vi "Slave.vi"() -> ()   [LabVIEW 2015]
uses:
  User Interface/Controls/Abort Test.ctl
  User Interface/Controls/Start Test.ctl
  User Interface/Controls/Configuration.ctl
  User Interface/Controls/Manual.ctl
  User Interface/Controls/Quit.ctl
  User Interface/UI Handler/Typedefs/Session Handle.ctl
  User Interface/UI Handler/UI Handler.lvclass
  Common/Circular Error Log/Typedefs/Session Handle.ctl
  Common/Circular Error Log/Circular Error Log.lvclass
  Tests/Controls/Test Config.ctl
  Tests/Controls/Gas Mixture.ctl
  CAN Communication/PAS/Typedefs/ADC Gains.ctl
  Tests/Controls/Filter Sequence.ctl
  Tests/Controls/Functional Test.ctl
  CAN Communication/PAS/Typedefs/Session Handle.ctl
  CAN Communication/PAS/PAS.lvclass
  Serial Device/Vaisala/Typedefs/Session Handle.ctl
  Serial Device/Vaisala/Vaisala.lvclass
  Tests/Controls/Test Info.ctl
  Serial Device/Environics/Typedefs/Session Handle.ctl
  Serial Device/Environics/Environics.lvclass
  Common/Buffers/Circular Buffer/Typedefs/Session Handle.ctl
  Common/Buffers/Circular Buffer/Circular Buffer.lvclass
  User Interface/UI Handler/Typedefs/References.ctl
  CAN Communication/PAS/Typedefs/Valves.ctl
  <vilib>/Utility/file.llb/Read Delimited Spreadsheet (string).vi
  Common/State Machine/State Machine.lvlib
  Common/Buffers/Snapshot/Snapshot.lvclass
  <vilib>/Analysis/NI_AALBase.lvlib
panel:
  in  "Quit":T1
  in  "Manual":T2
  in  "Configuration":T3
  in  "Start Test":T4
  in  "Abort Test":T5
  out "Samples Left":u16
  out "Filter Position":u8(knob) scale=1.0..12.0
  in  "Test":string
  out "PEL Temp":dbl caption="PEL Temp (C)" format="%.2f"
  out "PAS Temp":dbl caption="PAS Temp (C)" format="%.2f"
  out "Leak Rate":dbl caption="Leak Rate (PSI/s)" format="%.2f"
  out "Error?":bool
  out "Gas Stable?":bool
  out "Time Remaining":u32 caption="Time (s)"
  out "Moisture":dbl
  out "PPM":dbl caption="Actual PPM"
  out "Gas":string caption="Current Gas"
  in  "Broadcast":string
  out "exit":bool
  in  "Display":string
  out "Pressure":dbl caption="Gas Pressure (PSI)" format="%.2f"
  in  "Gas Sequence":i32(listbox)=-2
  in  "Message Log":string
  # "PAS Calibraton SLAVE"
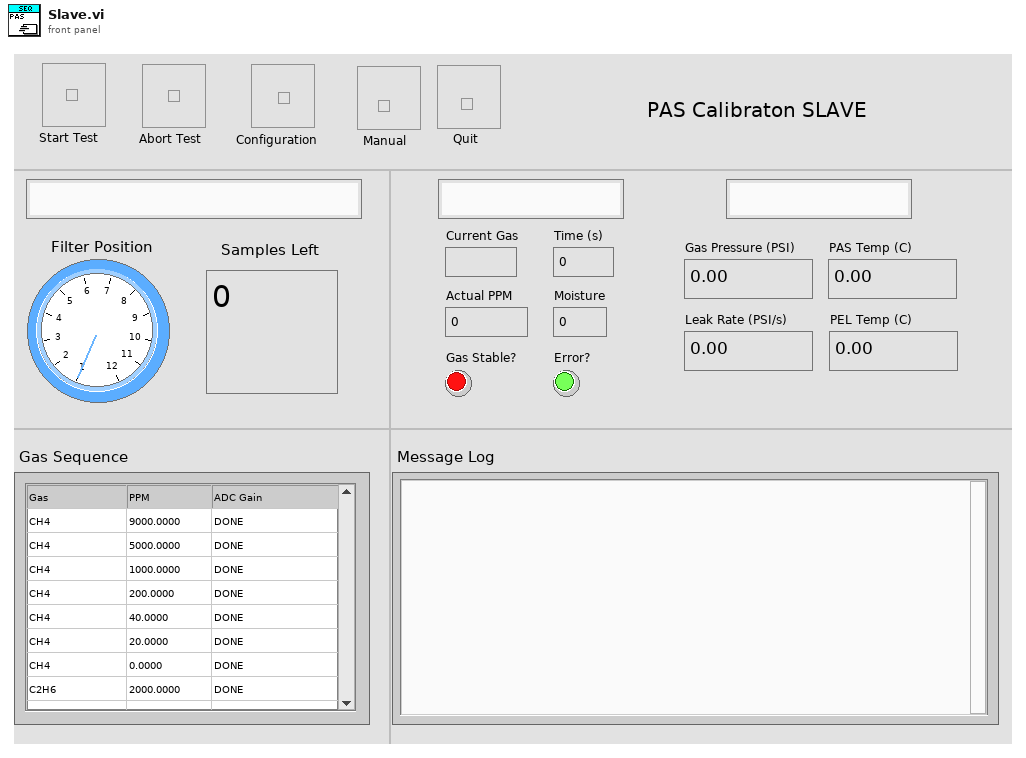
[diagram p1: front panel]
types:
  T1 = typedef "Quit.ctl" = bool
  T2 = typedef "Manual.ctl" = bool
  T3 = typedef "Configuration.ctl" = bool
  T4 = typedef "Start Test.ctl" = bool
  T5 = typedef "Abort Test.ctl" = bool
  T6 = enum8{"Enabled", "Disabled", "Disabled and Grayed Out"}
  T7 = typedef "UI Handler.lvclass/Session Handle.ctl" = refnum<data-value>
  T8 = typedef "Circular Error Log.lvclass/Session Handle.ctl" = refnum<data-value>
  T9 = typedef "Test Config.ctl" = cluster{"Chopper RPM":u16, "IR Power":u8, "Conc Tolerance":dbl, "Gas Stable Time":u16, "A-D Settle":u16, "Samples":u16, "Filter Time":u16, "Gas Mixtures":T10[], "Filter Sequences":T12[], "Functional Test":T13, "Initial Flow Rate":sgl, "Max Flow Rate":sgl}
  T10 = typedef "Gas Mixture.ctl" = cluster{"Gas":string, "PPM":dbl, "ADC Gains":T11}
  T11 = typedef "PAS.lvclass/ADC Gains.ctl" = u16
  T12 = typedef "Filter Sequence.ctl" = cluster{"Filter":u8, "Phase":dbl}
  T13 = typedef "Functional Test.ctl" = cluster{"Mic Test ON ADC Max":dbl, "Mic Test ON ADC Min":dbl, "Mic Test OFF ADC Max":dbl, "Mic Test OFF ADC Min":dbl, "Mic Test IC ADC Max":dbl, "Mic Test IC ADC Min":dbl, "IR Emitter ON ADC Max":dbl, "IR Emitter ON ADC Min":dbl, "IR Emitter OFF ADC Max":dbl, "IR Emitter OFF ADC Min":dbl}
  T14 = typedef "PAS.lvclass/Session Handle.ctl" = refnum<data-value>
  T15 = typedef "Vaisala.lvclass/Session Handle.ctl" = refnum<data-value>
  T16 = typedef "Test Info.ctl" = cluster{"Gas Counter":u16, "Filter Counter":u16, "ADC Samples":dbl[], "Gas Timeout":u16, "Notes":string, "Moisture":dbl, "PPM":dbl, "Mean":dbl, "STD":dbl, "Gas":string, "Pressure":dbl, "Temp":dbl, "Samples":u16, "Filter":u8, "Phase":dbl}
  T17 = typedef "Environics.lvclass/Session Handle.ctl" = refnum<data-value>
  T18 = typedef "Circular Buffer.lvclass/Session Handle.ctl" = refnum<data-value>
  T19 = cluster{"State":refnum<queue>, "UI Handler":T7, "Serial Number":string, "Error":T8, "Operator":string, "config path":path, "Test Config":T9, "PAS":T14, "Vaisala":T15, "Test Info":T16, "Test Results":string[][], "Environics":T17, "Cutoff":i32, "Root":path, "Circular Buffer":T18, "Zero Mean":dbl, "Zero Offsets":dbl[], "Results":T16[], "Blow Readings":cluster{"mean":dbl, "standard deviation":dbl}[], "Zero Readings":cluster{"mean":dbl, "standard deviation":dbl}[]}
  T20 = cluster{"Current Gas":string, "Actual PPM":dbl, "Moisture":dbl, "Time Remaining (s)":u32, "Stable?":bool, "Error?":bool}
  T21 = typedef "UI Handler.lvclass/References.ctl" = cluster{"Step":refnum<vi>, "Time":refnum<vi>, "Sequencer":refnum<vi>, "Log":refnum<vi>}
  T22 = cluster{"Serial Number Out":string, "Operator":string}
  T23 = typedef "PAS.lvclass/Valves.ctl" = u16
  T24 = typedef "Snapshot.lvclass/Session Handle.ctl" = refnum<data-value>
  T25 = typedef "User Configuration.ctl" = cluster{"Password":string, "cDAQ Name":string, "CAN Interface":string}
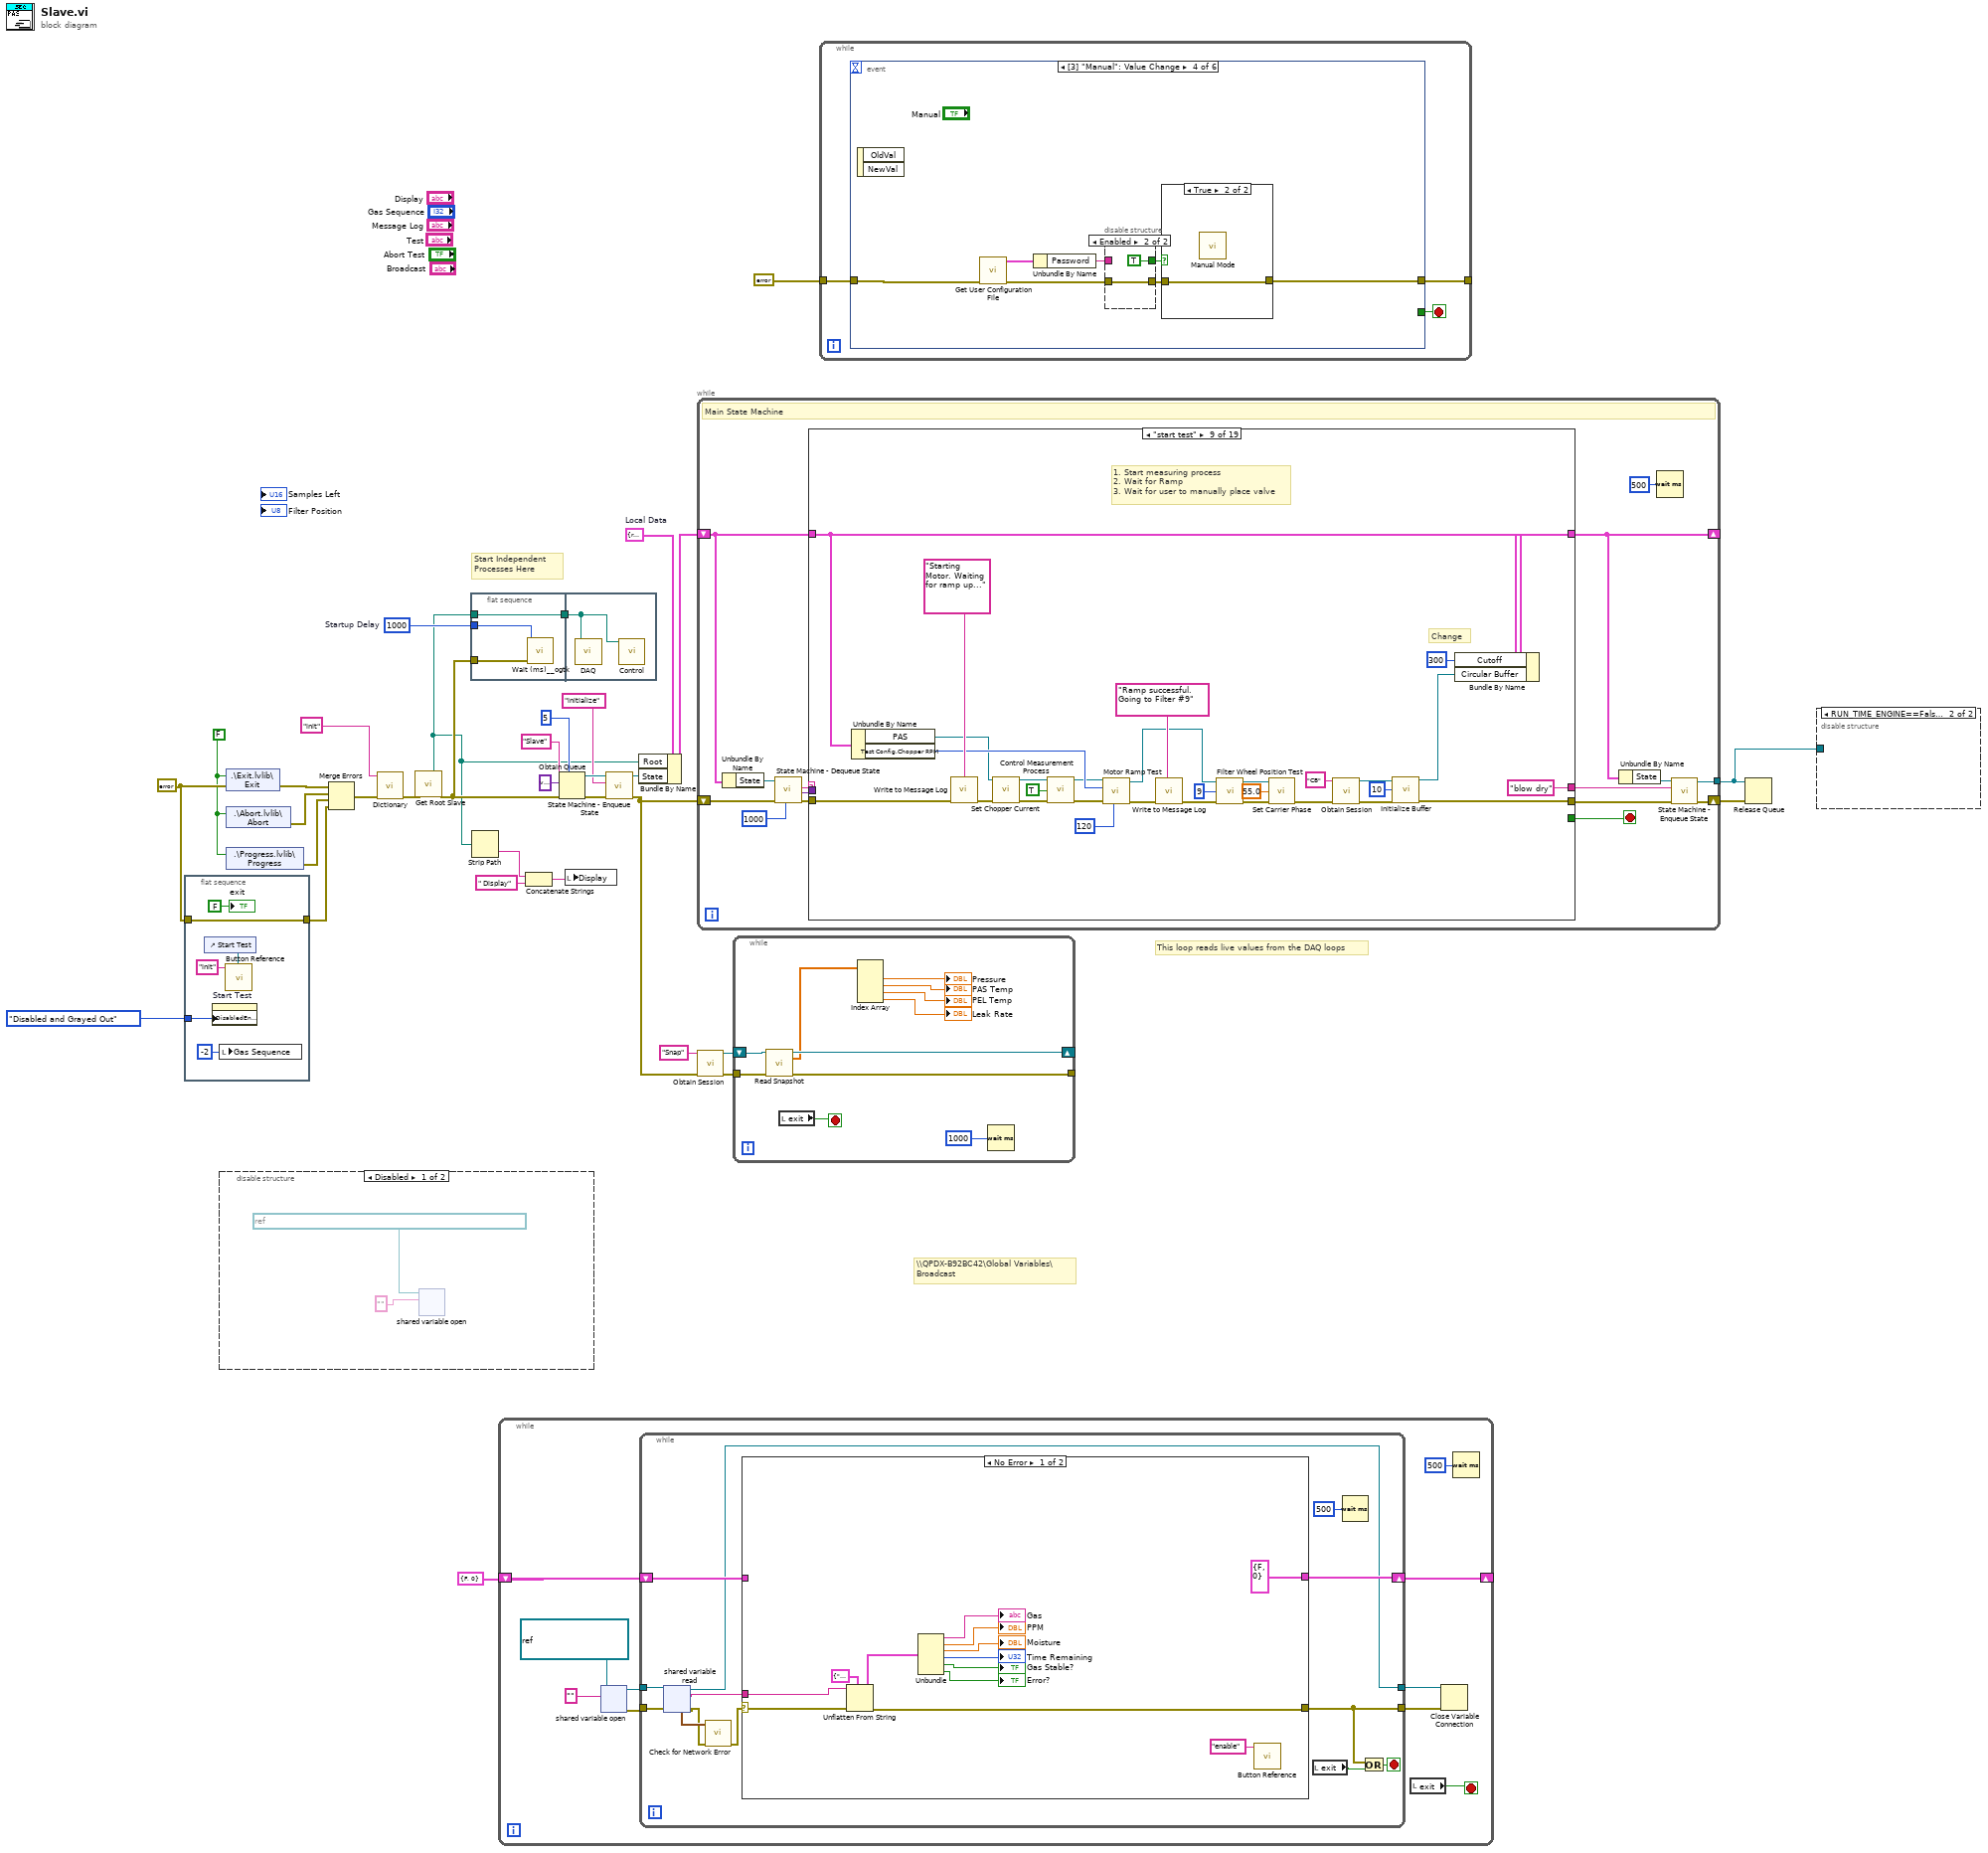
[diagram p0: block diagram]
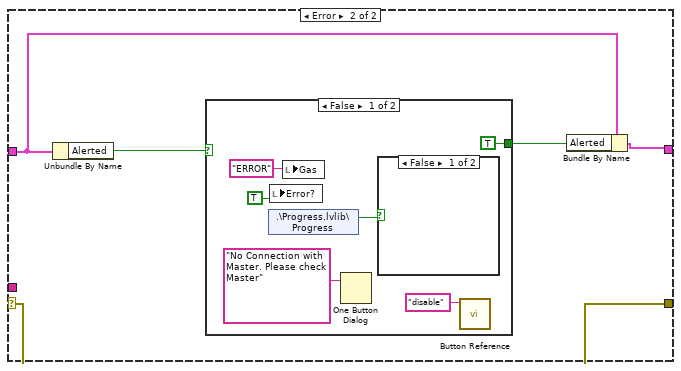
[diagram p3: hidden frame]
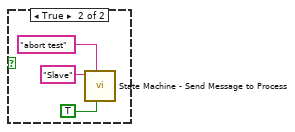
[diagram p4: hidden frame]
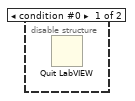
[diagram p6: hidden frame]
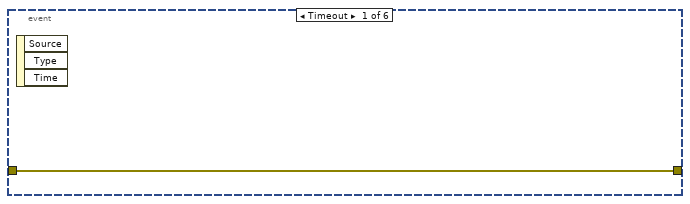
[diagram p7: hidden frame]
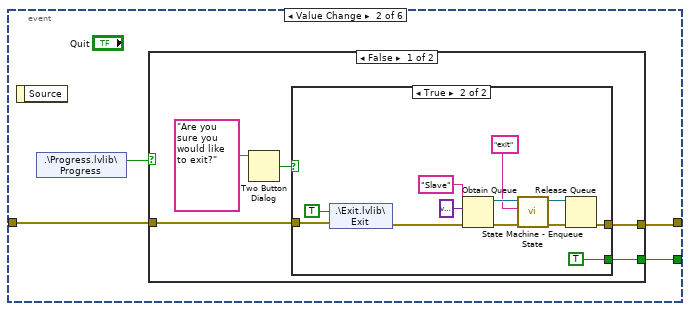
[diagram p8: hidden frame]
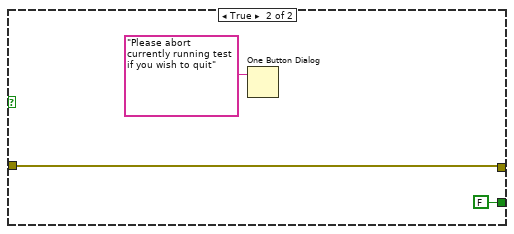
[diagram p10: hidden frame]
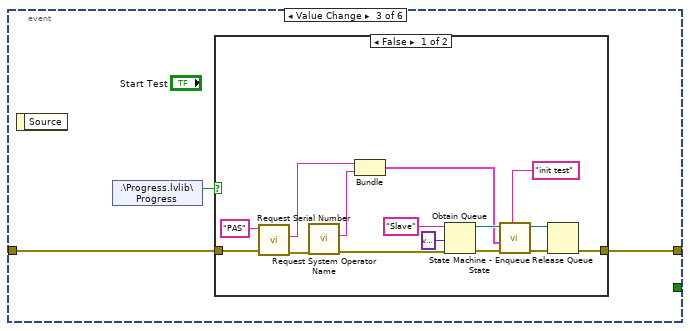
[diagram p11: hidden frame]
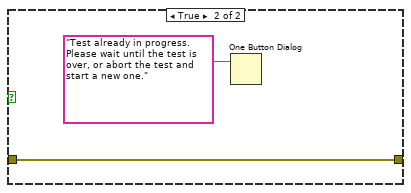
[diagram p12: hidden frame]
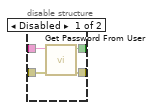
[diagram p13: hidden frame]
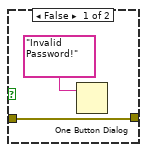
[diagram p14: hidden frame]
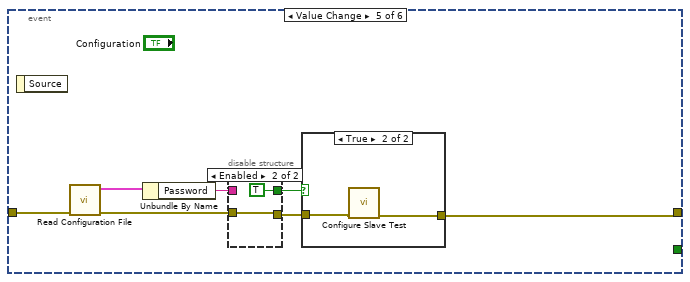
[diagram p15: hidden frame]
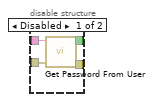
[diagram p16: hidden frame]
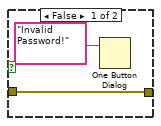
[diagram p17: hidden frame]
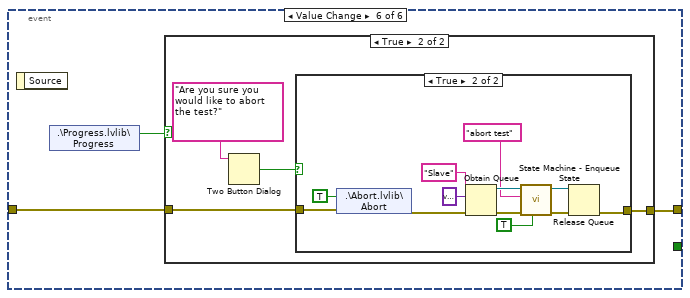
[diagram p18: hidden frame]
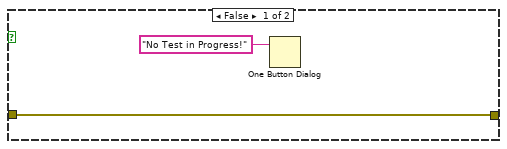
[diagram p19: hidden frame]
diagram:
  w1 = FALSE ("Exit")
  w25 = u32 1000  # Startup Delay
  w15 = errorcluster {"status"=FALSE, "code"=0, "source"=""} ("error in (no error)")
  w28 = T19 {"State"=refnum, "UI Handler"=refnum, "Serial Number"="", "Error"=refnum, "Operator"="", "config path"=path "", "Test Config"={"Chopper RPM"=140, "IR Power"=5, "Conc Tolerance"=0.0, "Gas Stable Time"=0, "A-D Settle"=0, "Samples"=0, "Filter Time"=0, "Gas Mixtures"=[], "Filter Sequences"=[], "Functional Test"={"Mic Test ON ADC Max"=0.0, "Mic Test ON ADC Min"=0.0, "Mic Test OFF ADC Max"=0.0, "Mic Test OFF ADC Min"=0.0, "Mic Test IC ADC Max"=0.0, "Mic Test IC ADC Min"=0.0, "IR Emitter ON ADC Max"=0.0, "IR Emitter ON ADC Min"=0.0, "IR Emitter OFF ADC Max"=0.0, "IR Emitter OFF ADC Min"=0.0}, "Initial Flow Rate"=0.0, "Max Flow Rate"=0.0}, "PAS"=refnum, "Vaisala"=refnum, "Test Info"={"Gas Counter"=0, "Filter Counter"=0, "ADC Samples"=[], "Gas Timeout"=0, "Notes"="", "Moisture"=0.0, "PPM"=0.0, "Mean"=0.0, "STD"=0.0, "Gas"="", "Pressure"=0.0, "Temp"=0.0, "Samples"=0, "Filter"=0, "Phase"=0.0}, "Test Results"=[], "Environics"=refnum, "Cutoff"=0, "Root"=path "", "Circular Buffer"=refnum, "Zero Mean"=0.0, "Zero Offsets"=[], "Results"=[], "Blow Readings"=[], "Zero Readings"=[]}  # Local Data
  # "\\\\QPDX-B92BC42\\Global Variables\\\nBroadcast"
  # "This loop reads live values from the DAQ loops"
  # "Start Independent\nProcesses Here"
  n1 = flat-sequence {
    tunnel: w15 -> [w39]
    tunnel: [w39] -> w14
    tunnel: T6."Disabled and Grayed Out" ("Disabled") -> [w36]
    frame #0 {
      n2 = control-ref of="Start Test"() -> (w37:refnum<vi>)
      n3 = property on="Start Test" class="Bool"("DisabledEnum"=w36) -> ()  [unwired: 2 in, 2 out]
      n4 = local write "Gas Sequence"(-2 ("Gas Sequence")) -> ()
      n5 = call "Button Reference.vi"("Ref In"=w37, "Command"="init") -> ()  [unwired: 9 in, 1 out]
      "exit" <- FALSE ("exit")
    }
  }
  n6 = disable-structure shown="Disabled" {
    frame Disabled {
      n7 = shared-variable-open(refnum<k21> "ni.var.psp://QPDX-B92BC42/Global Variables/Broadcast" ("shared variable refnum in"), "") -> ()  [unwired: 2 in, 2 out]
    }
    frame Enabled {
    }
  }
  n8 = shared-variable ".\\Exit.lvlib\\Exit"(w1, error in=w15) -> (error out=w23:errorcluster)
  n9 = shared-variable ".\\Abort.lvlib\\Abort"(w1) -> (error out=w24:errorcluster)  [unwired: 1 in]
  n10 = shared-variable ".\\Progress.lvlib\\Progress"(w1) -> (error out=w20:errorcluster)  [unwired: 1 in]
  n11 = Merge Errors(w23, w24, w20, w14) -> (w4:errorcluster)
  n12 = call "Dictionary.vi"("error in"=w4, "Command"="init") -> ("error out"=w3:errorcluster)  [unwired: 8 in, 1 out]
  n13 = call "Get Root Slave.vi"("error in (no error)"=w3) -> ("error out"=w10:errorcluster, "Root"=w5:path)  [unwired: 9 in]
  n14 = flat-sequence {
    tunnel: w10 -> [w43]
    tunnel: w25 -> [w45]
    tunnel: w5 -> [w44]
    tunnel: [w44] -> w9
    tunnel: w9 -> [w46]
    frame #0 {
      n15 = call <userlib>:"Wait (ms)__ogtk.vi"("error in (no error)"=w43, "milliseconds to wait"=w45) -> ()  [unwired: 8 in, 2 out]
    }
    frame #1 {
      n16 = call "DAQ.vi"("Folder"=w46) -> ()  [unwired: 11 in]
      n17 = call "Control.vi"("Root"=w46) -> ()  [unwired: 11 in]
    }
  }
  n18 = Strip Path(path=w5) -> (name=w8:string)  [unwired: 1 out]
  n19 = while {
    shift-right: [w53] -> _
    shift-left: cluster{"Alerted":bool, "Packets Lost":i32} {"Alerted"=FALSE, "Packets Lost"=0} -> [w54]
    stop <- w56 stop-if-true
    n20 = shared-variable-open(refnum<k21> "ni.var.psp://localhost/Global Variables/Broadcast" ("shared variable refnum in"), "") -> (w50:refnum<k21>, w51:errorcluster)  [unwired: 2 in]
    n21 = while {
      tunnel: w50 -> [w63]
      tunnel: [w61] -> w48
      tunnel: w51 -> [w64]
      tunnel: [w68] -> w49
      shift-right: [w65] -> w53
      shift-left: w54 -> [w66]
      stop <- w69 stop-if-true
      # "UDP Receiver Loop"
      n22 = shared-variable-read(w63, w64) -> (w61:refnum<k21>, w59:errorcluster, w62:string, w60:timestamp)
      n23 = call "Check for Network Error.vi"("error in (no error)"=w59, "Time Stamp"=w60) -> ("error out"=w58:errorcluster)  [unwired: 9 in]
      n24 = case shown="No Error" w58 {
        selector: w58 -> [w82 w84]
        tunnel: w62 -> [w81 _]
        tunnel: [w79 w84] -> w68
        tunnel: w66 -> [_ w85]
        tunnel: [cluster{"Alerted":bool, "Packets Lost":i32} {"Alerted"=FALSE, "Packets Lost"=0} w87] -> w65
        frame No Error {
          # "Sender sent data. Update the chart value."
          n25 = Unflatten From String(type=T20 {"Current Gas"="", "Actual PPM"=0.0, "Moisture"=0.0, "Time Remaining (s)"=0, "Stable?"=FALSE, "Error?"=FALSE} ("output cluster"), binary string=w81, error in (no error)=w82) -> (value=w78:T20, error out=w79:errorcluster)  [unwired: 2 in, 1 out]
          n26 = Unbundle(w78) -> ("Current Gas"=→"Gas":string, "Actual PPM"=→"PPM":dbl, "Moisture"=→"Moisture":dbl, "Time Remaining (s)"=→"Time Remaining":u32, "Stable?"=→"Gas Stable?":bool, "Error?"=→"Error?":bool)
          n27 = call "Button Reference.vi"("Command"="enable") -> ()  [unwired: 10 in, 1 out]
        }
        frame Error {
          # "Sender did not send data. Ignore timeout error and keep waiting."
          n28 = Unbundle By Name(w85) -> ("Alerted"=w86:bool)
          n29 = case shown="False" w86 {
            selector: w86 -> [_ w97]
            tunnel: [TRUE w97] -> w83
            frame False {
              n30 = shared-variable ".\\Progress.lvlib\\Progress"() -> (w93:bool)  [unwired: 1 in, 1 out]
              n31 = local write "Error?"(TRUE ("Error?")) -> ()
              n32 = local write "Gas"("ERROR" ("Gas")) -> ()
              n33 = One Button Dialog(message="No Connection with Master. Please check Master") -> ()  [unwired: 1 in, 1 out]
              n34 = case shown="False" w93 {
                frame False {
                }
                frame True {
                  n35 = call "State Machine - Send Message to Process.vi"("Front?"=TRUE, "State"="abort test", "Process Name"="Slave") -> ()  [unwired: 8 in, 1 out]
                }
              }
              n36 = call "Button Reference.vi"("Command"="disable") -> ()  [unwired: 10 in, 1 out]
            }
            frame True {
            }
          }
          n37 = Bundle By Name(cluster=w85, "Alerted"=w83) -> (w87:cluster{"Alerted":bool, "Packets Lost":i32})
        }
      }
      n38 = local read "exit"() -> (w67:bool)
      n39 = Wait (ms)(milliseconds to wait=u32 500) -> ()  [unwired: 1 out]
      n40 = Or(x=w68, y=w67) -> (x .or. y?=w69:bool)
    }
    n41 = local read "exit"() -> (w56:bool)
    n42 = Close Variable Connection(8:w49, 11:w48) -> ()  [unwired: 1 out]
    n43 = Wait (ms)(milliseconds to wait=u32 500) -> ()  [unwired: 1 out]
  }
  n44 = Concatenate Strings(w8, " Display" ("string")) -> (w6:string)
  n45 = Obtain Queue(max queue size (-1, unlimited)=5, name (unnamed)="Slave", element data type=variant, error in (no error)=w10) -> (queue out=w30:refnum<queue>, error out=w31:errorcluster)  [unwired: 1 in, 1 out]
  n46 = local write "Display"(w6) -> ()
  n47 = call "State Machine - Enqueue State.vi"("error in (no error)"=w31, "State"="initialize", "Queue In"=w30) -> ("error out"=w18:errorcluster, "Queue Out"=w27:refnum<queue>)  [unwired: 7 in]
  n48 = Bundle By Name(cluster=w28, "Root"=w5, "State"=w27) -> (w26:T19)
  n49 = while "Main State Machine" {
    shift-right: [w109] -> w21
    shift-left: w18 -> [w112]
    shift-right: [w100] -> _
    shift-left: w26 -> [w103]
    tunnel: [w98] -> w13
    stop <- w105 stop-if-true
    # "Main State Machine"
    n50 = Unbundle By Name(w103) -> ("State"=w102:refnum<queue>)
    n51 = call "State Machine - Dequeue State.vi"("Timeout"=1000, "error in (no error)"=w112, "Queue In"=w102) -> ("error out"=w111:errorcluster, "Data"=w99:variant, "State"=w110:string)  [unwired: 4 in, 2 out]
    n52 = case shown="\"start test\"" w110 {
      tunnel: w111 -> [w124 w150 w164 w188 w190 _ w232 w266 w288 w302 w335 w377 w409 w443 w497 w516 w546 w555 w580]
      tunnel: [w138 w147 w168 w188 w190 w195 w211 w261 w281 w306 w330 w381 w403 w439 w493 w512 w539 w551 w577] -> w108
      tunnel: ["init local" ("State") _ _ _ _ _ w226 "start test" ("Error String") "blow dry" ("Error String") w307 w343 "filter" ("Error String") w410 w440 "start mix" ("Error String") "record result" ("Error String") "filter" ("Error String") _ _] -> w107
      tunnel: [_ _ _ _ _ TRUE _ _ _ _ _ _ _ _ _ _ _ _ _] -> w105
      tunnel: w103 -> [w114 w157 w161 w187 w189 w198 w229 w265 w287 w303 w342 w399 w408 w435 w499 w520 w549 w569 w576]
      tunnel: [w143 w157 w166 w187 w189 w198 w230 w264 w286 w303 w336 w398 w408 w434 w499 w519 w548 w569 w576] -> w100
      tunnel: w99 -> [_ _ _ _ _ _ w231 _ _ _ _ _ _ _ _ _ _ _ _]
      frame "initialize" {
        # "1. Setup UI Handler\n2. Setup Error Logger\n3. Get list of gases"
        n53 = Unbundle By Name(w114) -> ("Root"=w113:path)
        n54 = Build Path(base path=w113, name or relative path="Configuration\\Gases.txt") -> (appended path=w123:path)
        n55 = call-poly <vilib>:"Read Delimited Spreadsheet.vi"("file path (dialog if empty)"=w123, "error in (no error)"=w124, "delimiter (\\t)"="\r") -> ("all rows"=w117:string[][], "error out"=w121:errorcluster)  [unwired: 7 in, 4 out]
        n56 = Index Array(array=w117, index (col)=0 ("disabled index (col)")) -> (element=w116:string[])  [unwired: 1 in]
        n57 = control-ref of="Gas Sequence"() -> (w128:refnum<vi>)
        n58 = call "Dictionary.vi"("error in"=w121, "Value"=w116, "Key"="Gas", "Command"="set") -> ("error out"=w118:errorcluster)  [unwired: 6 in, 1 out]
        n59 = control-ref of="Message Log"() -> (w127:refnum<vi>)
        n60 = Bundle By Name(cluster=T21 {"Step"=refnum, "Time"=refnum, "Sequencer"=refnum, "Log"=refnum} ("References"), "Sequencer"=w128, "Log"=w127) -> (w126:T21)
        n61 = call "Obtain Session.vi"("Session  Name ()"="UIH", "error in (no error)"=w118) -> ("Session Handle"=w130:T7, "error out"=w133:errorcluster)  [unwired: 12 in]
        n62 = call "Initialize References.vi"("Session Handle in"=w130, "References"=w126, "error in (no error)"=w133) -> ("Session Handle out"=w131:T7, "error out"=w132:errorcluster)  [unwired: 11 in]
        n63 = Build Path(base path=w113, name or relative path="Error\\error.txt") -> (appended path=w135:path)
        n64 = call "Obtain Session.vi"("Session  Name ()"="Error", "error in (no error)"=w132) -> ("Session Handle"=w140:T8, "error out"=w141:errorcluster)  [unwired: 12 in]
        n65 = call "Initialize Error Log.vi"("Session Handle in"=w140, "Error Path"=w135, "Max File Size"=i64 5000000, "error in (no error)"=w141) -> ("Session Handle out"=w137:T8, "error out"=w138:errorcluster)  [unwired: 10 in]
        n66 = Bundle By Name(cluster=w114, "UI Handler"=w131, "Error"=w137) -> (w143:T19)
      }
      frame "init local" {
        w146 = 0.0 ("Test Pressure (PSI)")
        # "1. Set Filter Position and Samples Remaining to 20\n2. Clear Listbox and Log\n3. Set Live Display and Test to values \n4. Set Live Display values to 0"
        n67 = call "Initialize Message Log.vi"("error in (no error)"=w150) -> ("error out"=w156:errorcluster)  [unwired: 10 in]
        n68 = call "Clear Sequence.vi"("error in (no error)"=w156) -> ("error out"=w153:errorcluster)  [unwired: 10 in]
        n69 = call "Write to Message Log.vi"("error in (no error)"=w153, "Message"="PAS Calibration Started...") -> ("error out"=w145:errorcluster)  [unwired: 9 in]
        n70 = property on="Test" class="Str"(error in=w145, "Value"="No Test In Progress..." ("Test")) -> (error out=w149:errorcluster)  [unwired: 1 in, 1 out]
        n71 = property on="Broadcast" class="Str"(error in=w149, "Text.Text"="Broadcast Data...") -> (error out=w147:errorcluster)  [unwired: 1 in, 1 out]
        n72 = local write "Pressure"(w146) -> ()
        n73 = local write "PAS Temp"(w146) -> ()
        n74 = local write "PEL Temp"(w146) -> ()
        n75 = local write "Leak Rate"(w146) -> ()
        n76 = local write "Filter Position"(u8 0 ("Filter Position")) -> ()
        n77 = local write "Samples Left"(u16 0 ("Samples Left")) -> ()
      }
      frame "error" {
        # "1. If a test was in progress..."
        n78 = call "Data Changed.vi"("Data"=w164) -> ("Changed?"=w163:bool)  [unwired: 10 in]
        n79 = case shown="True" w163 {
          tunnel: [w169 w173] -> w160
          tunnel: w164 -> [w170 w174]
          frame False {
            n80 = Unbundle By Name(w170) -> ("source"=w171:string)
            n81 = Concatenate Strings("Error: " ("string"), w171) -> (w169:string)
          }
          frame True {
            n82 = Unbundle By Name(w174) -> ("source"=w175:string)
            n83 = Concatenate Strings("Error: " ("string"), w175) -> (w173:string)
            n84 = call "Dialog Box.vi"("Serial Number"=w173) -> ()  [unwired: 10 in, 1 out]
          }
        }
        n85 = Unbundle By Name(w161) -> ("Error"=w162:T8)
        n86 = call "Write to Message Log.vi"("Message"=w160) -> ()  [unwired: 10 in, 1 out]
        n87 = shared-variable ".\\Progress.lvlib\\Progress"() -> (w165:bool)  [unwired: 1 in, 1 out]
        n88 = call "Write Error Log.vi"("Session Handle in"=w162, "Process Name"="Main", "Data"=w160) -> ()  [unwired: 11 in, 2 out]
        n89 = case shown="True" w165 {
          tunnel: w161 -> [w177 w181]
          tunnel: [w177 w181] -> w166
          tunnel: w160 -> [_ _]
          frame False {
          }
          frame True {
            n90 = shared-variable ".\\Progress.lvlib\\Progress"(FALSE ("Progress")) -> (error out=w184:errorcluster)  [unwired: 1 in]
            n91 = call "Initialize Hardware.vi"("error in"=w184) -> ("error out"=w180:errorcluster)  [unwired: 10 in]
            n92 = local write "Test"("Test Error..." ("Test")) -> ()
            n93 = call "File Tracker.vi"("Command"="close", "error in (no error)"=w180) -> ("error out"=w179:errorcluster)  [unwired: 8 in, 1 out]
            n94 = flat-sequence {
              tunnel: "Error occured. Please see log for details. The test has been aborted" -> [w186]
              tunnel: w179 -> [_]
              frame #0 {
                n95 = One Button Dialog(message=w186) -> ()  [unwired: 1 in, 1 out]
              }
            }
          }
        }
        n96 = Unbundle By Name(w166) -> ("State"=w167:refnum<queue>)
        n97 = Wait (ms)(milliseconds to wait=u32 1000) -> ()  [unwired: 1 out]
        n98 = Flush Queue(queue=w167) -> (error out=w168:errorcluster)  [unwired: 1 in, 2 out]
      }
      frame Default {
      }
      frame "idle" {
      }
      frame "exit" {
        # "1. Clean up all references\n2. Exit commands to Datalogger"
        n99 = Unbundle By Name(w198) -> ("UI Handler"=w197:T7)
        n100 = call "Release Session.vi"("Session Handle"=w197) -> ("error out"=w193:errorcluster)  [unwired: 14 in]
        n101 = call "Write to Message Log.vi"("error in (no error)"=w193, "Message"="Initializing Hardware Before Exiting...") -> ("error out"=w192:errorcluster)  [unwired: 9 in]
        n102 = call "Initialize Hardware.vi"("error in"=w192) -> ("error out"=w191:errorcluster)  [unwired: 10 in]
        n103 = local write "exit"(TRUE ("exit")) -> ()
        n104 = flat-sequence {
          tunnel: [w200] -> w195
          tunnel: w191 -> [_]
          frame #0 {
            n105 = call "State Machine - Send Message to Process.vi"("Front?"=TRUE, "State"="exit", "Process Name"="DAQ") -> ("error out"=w201:errorcluster)  [unwired: 8 in]
            n106 = call "State Machine - Send Message to Process.vi"("Front?"=TRUE, "State"="exit", "error in (no error)"=w201, "Process Name"="Control") -> ("error out"=w200:errorcluster)  [unwired: 7 in]
          }
        }
      }
      frame "init test" {
        # "1. Initialize all Hardware\n2. Store Serial Number\n3. Send start command to logger\n4.. Proceed to Test"
        n107 = Variant To Data(error in=w232, type=T22 {"Serial Number Out"="", "Operator"=""} ("cluster"), Variant=w231) -> (data=w222:T22, error out=w221:errorcluster)
        n108 = call "Get Slave Configuration File from User.vi"("error in"=w221) -> ("error out"=w220:errorcluster, "Test Config"=w219:T9, "selected path"=w215:path)  [unwired: 7 in, 1 out]
        n109 = disable-structure shown="Enabled" {
          disable-tunnel: [w236 w238] -> w225
          disable-tunnel: [w235 TRUE ("Go on?")] -> w224
          disable-tunnel: w220 -> [w234 w238]
          disable-tunnel: w219 -> [w233 _]
          frame Disabled {
            n110 = call "PAS Functional Test.vi"("error in (no error)"=w234, "Test Config"=w233) -> ("Error Out"=w236:errorcluster, "Go on?"=w235:bool)  [unwired: 8 in]
          }
          frame Enabled {
          }
        }
        n111 = local write "Test"("Test In Progress..." ("Test")) -> ()
        n112 = case shown="False" w224 {
          tunnel: [w244 w247] -> w211
          tunnel: w225 -> [w244 w251]
          tunnel: [w239 w246] -> w212
          tunnel: [_ TRUE ("Progress")] -> w223
          tunnel: w222 -> [w243 w255]
          tunnel: [w241 w253] -> w216
          tunnel: w219 -> [w239 w246]
          tunnel: [w242 w254] -> w217
          tunnel: w215 -> [w240 w252]
          tunnel: [w240 w252] -> w214
          frame False {
            n113 = Unbundle By Name(w243) -> ("Operator"=w242:string, "Serial Number Out"=w241:string)
          }
          frame True {
            n114 = Unbundle By Name(w255) -> ("Operator"=w254:string, "Serial Number Out"=w253:string)
            n115 = call "Write to Message Log.vi"("error in (no error)"=w251, "Message"="Test Starting...") -> ("error out"=w250:errorcluster)  [unwired: 9 in]
            n116 = call "Write to Message Log.vi"("error in (no error)"=w250, "Message"="Initializing Hardware...") -> ("error out"=w260:errorcluster)  [unwired: 9 in]
            n117 = call "Initialize Hardware.vi"("error in"=w260) -> ("error out"=w256:errorcluster)  [unwired: 10 in]
            n118 = shared-variable ".\\Progress.lvlib\\Progress"(TRUE ("Progress"), error in=w256) -> (error out=w248:errorcluster)
            n119 = call "Test Tracker.vi"("Command"="init", "Test Config"=w246) -> ()  [unwired: 6 in, 4 out]
            n120 = call "Write Gas Sequence.vi"("error in (no error)"=w248, "Test Config"=w246) -> ("error out"=w247:errorcluster)  [unwired: 9 in]
          }
        }
        n121 = Bundle By Name(cluster=w229, "Test Info"=T16 {"Gas Counter"=0, "Filter Counter"=0, "ADC Samples"=[], "Gas Timeout"=0, "Notes"="", "Moisture"=0.0, "PPM"=0.0, "Mean"=0.0, "STD"=0.0, "Gas"="", "Pressure"=0.0, "Temp"=0.0, "Samples"=0, "Filter"=0, "Phase"=0.0}, "Operator"=w217, "Serial Number"=w216, "config path"=w214, "Test Config"=w212, "Zero Readings"=cluster{"mean":dbl, "standard deviation":dbl}[] [], "Results"=T16[] []) -> (w230:T19)
        n122 = Select(t="get refs" ("Error String"), s=w223, f="idle" ("Error String")) -> (s? t:f=w226:string)
      }
      frame "get refs" {
        # "1. Get References to PAS"
        n123 = call "Obtain Session.vi"("Session  Name ()"="PAS", "error in (no error)"=w266) -> ("Session Handle"=w263:T14, "error out"=w261:errorcluster)  [unwired: 12 in]
        n124 = Bundle By Name(cluster=w265, "PAS"=w263) -> (w264:T19)
      }
      frame "start test" {
        # "Change"
        # "1. Start measuring process\n2. Wait for Ramp\n3. Wait for user to manually place valve"
        n125 = Unbundle By Name(w287) -> ("PAS"=w271:T14, "Test Config.Chopper RPM"=w296:u16)
        n126 = call "Write to Message Log.vi"("error in (no error)"=w288, "Message"="Starting Motor. Waiting for ramp up...") -> ("error out"=w268:errorcluster)  [unwired: 9 in]
        n127 = call "Set Chopper Current.vi"("Session Handle in"=w271, "error in (no error)"=w268) -> ("Session Handle out"=w270:T14, "error out"=w269:errorcluster)  [unwired: 11 in, 1 out]
        n128 = call "Control Measurement Process.vi"("Session Handle in"=w270, "Start?"=TRUE, "error in (no error)"=w269) -> ("Session Handle out"=w290:T14, "error out"=w291:errorcluster)  [unwired: 9 in, 2 out]
        n129 = call "Motor Ramp Test.vi"("Timeout"=u32 120, "error in (no error)"=w291, "RPM"=w296, "Session Handle in"=w290) -> ("error out"=w294:errorcluster, "Session Handle out"=w277:T14)  [unwired: 5 in, 1 out]
        n130 = call "Write to Message Log.vi"("error in (no error)"=w294, "Message"="Ramp successful. Going to Filter #9") -> ("error out"=w279:errorcluster)  [unwired: 9 in]
        n131 = call "Filter Wheel Position Test.vi"("error in (no error)"=w279, "Position"=u8 9, "Session Handle in"=w277) -> ("error out"=w276:errorcluster, "Session Handle out"=w275:T14)  [unwired: 6 in, 1 out]
        n132 = call "Set Carrier Phase.vi"("Session Handle in"=w275, "Phase"=55.0, "error in (no error)"=w276) -> ("error out"=w273:errorcluster)  [unwired: 10 in, 2 out]
        n133 = call "Obtain Session.vi"("Session  Name ()"="CB", "error in (no error)"=w273) -> ("Session Handle"=w283:T18, "error out"=w284:errorcluster)  [unwired: 12 in]
        n134 = call "Initialize Buffer.vi"("Session Handle in"=w283, "Size"=u16 10, "error in (no error)"=w284) -> ("Session Handle out"=w280:T18, "error out"=w281:errorcluster)  [unwired: 11 in]
        n135 = Bundle By Name(cluster=w287, "Cutoff"=300, "Circular Buffer"=w280) -> (w286:T19)
      }
      frame "blow dry" {
        n136 = call "Dialog Box.vi"("error in (no error)"=w302, "Serial Number"="Beginning the Blow Dry process. Please turn the 3 Way Valve to the correct position...") -> ("error out"=w300:errorcluster)  [unwired: 9 in]
        n137 = call "File Tracker.vi"("Command"="new", "error in (no error)"=w300) -> ("error out"=w299:errorcluster)  [unwired: 8 in, 1 out]
        n138 = call "Write to Message Log.vi"("error in (no error)"=w299, "Message"="Conducting Blow Dry Test...") -> ("error out"=w304:errorcluster)  [unwired: 9 in]
        n139 = Unbundle By Name(w303) -> ("Circular Buffer"=w309:T18, "PAS"=w308:T14)
        n140 = disable-structure shown="Enabled" {
          disable-tunnel: w309 -> [w318 _]
          disable-tunnel: w308 -> [w317 _]
          disable-tunnel: [w313 "zero offset" ("State")] -> w307
          disable-tunnel: [w312 w326] -> w306
          disable-tunnel: w304 -> [w311 w326]
          frame Disabled {
            # "todo: add config"
            n141 = call "Blow Dry Test.vi"("Tol"=10000.0, "error in (no error)"=w311, "PAS"=w317, "Circular Buffer"=w318) -> ("error out"=w315:errorcluster, "Aborted?"=w314:bool, "Test Reading"=w310:cluster{"mean":dbl, "standard deviation":dbl})  [unwired: 4 in, 1 out]
            n142 = case shown="False" w314 {
              tunnel: w315 -> [w321 w323]
              tunnel: [w320 w323] -> w312
              tunnel: ["zero offset" ("State") "abort test" ("State")] -> w313
              tunnel: w310 -> [_ _]
              frame False {
                n143 = call "Write to Message Log.vi"("error in (no error)"=w321, "Message"="Blow Dry Test Succeeded") -> ("error out"=w320:errorcluster)  [unwired: 9 in]
              }
              frame True {
              }
            }
          }
          frame Enabled {
          }
        }
      }
      frame "zero offset" {
        # "todo: add config"
        n144 = Unbundle By Name(w342) -> ("PAS"=w341:T14)
        n145 = call "Flush Gas.vi"("Display UI?"=TRUE, "error in (no error)"=w335, "PAS"=w341) -> ("error out"=w333:errorcluster, "PAS Out"=w339:T14)  [unwired: 7 in]
        n146 = call "Write to Message Log.vi"("error in (no error)"=w333, "Message"="Conducting Zero Offset Test...") -> ("error out"=w332:errorcluster)  [unwired: 9 in]
        n147 = call "Zero Offset Test.vi"("Tol"=10000.0, "error in (no error)"=w332, "PAS"=w339) -> ("error out"=w345:errorcluster, "Aborted?"=w344:bool, "Success?"=w338:bool, "Readings"=w337:cluster{"mean":dbl, "standard deviation":dbl}[])  [unwired: 5 in]
        n148 = case shown="False" w344 {
          tunnel: w345 -> [w350 w361]
          tunnel: [w349 w361] -> w331
          tunnel: [w351 "abort test" ("State")] -> w343
          tunnel: [w346 _] -> w329
          tunnel: w338 -> [w348 _]
          tunnel: w337 -> [w347 _]
          frame False {
            n149 = case shown="True" w348 {
              tunnel: [_ "wait mix" ("State")] -> w351
              tunnel: w350 -> [w354 w359]
              tunnel: [w353 w358] -> w349
              tunnel: [w355 w356] -> w346
              tunnel: w347 -> [w355 w356]
              frame False {
                n150 = Merge Errors(w354, errorcluster {"status"=TRUE, "code"=781, "source"="Inconsistent ADC Readings for Zero Offset Test"} ("error in")) -> (w353:errorcluster)
              }
              frame True {
                n151 = call "Write to Message Log.vi"("error in (no error)"=w359, "Message"="Zero Offset Test Succeeded. Starting test...") -> ("error out"=w358:errorcluster)  [unwired: 9 in]
              }
            }
          }
          frame True {
          }
        }
        n152 = Bundle By Name(cluster=w342, "Zero Readings"=w329) -> (w336:T19)
        n153 = call "File Tracker.vi"("Command"="write zero", "error in (no error)"=w331, "Readings"=w329) -> ("error out"=w330:errorcluster)  [unwired: 7 in, 1 out]
      }
      frame "start mix" {
        w392 = T23 18 items=["PV1"=17, "PV2"=18, "PV3"=19, "PV4"=20] ("Valves")
        w390 = T23 17 items=["PV1"=17, "PV2"=18, "PV3"=19, "PV4"=20] ("Valves")
        # "When energizing - PV2 wait PV1\nWhen deenergizing - PV1 wait PV2"
        # "1. Update Gas in Test Info\n2. Set PV1, PV2 ON\n3. Set ADC Gain\n4. Turn on SV1 and GV1 to let the gas pass through\n5. Record PPM and Moisture"
        n154 = Unbundle By Name(w399) -> ("Test Info"=w402:T16, "Test Config.Samples"=w371:u16, "Test Config.Gas Mixtures"=w401:T10[], "PAS"=w383:T14)
        n155 = call "NI DAQ Channels.vi"("Control"=TRUE, "Channel"="SV1", "error in (no error)"=w377) -> ("error out"=w375:errorcluster)  [unwired: 7 in, 1 out]
        n156 = call "Test Tracker.vi"("Command"="get gas", "error in (no error)"=w375) -> ("error out"=w374:errorcluster, "Gas Index"=w372:i32)  [unwired: 6 in, 2 out]
        n157 = local write "Gas Sequence"(w372) -> ()
        n158 = local write "Samples Left"(w371) -> ()
        n159 = call "Control Valve.vi"("Session Handle in"=w383, "Valves"=w390, "Energize?"=FALSE, "error in (no error)"=w374) -> ("Session Handle out"=w387:T14, "error out"=w388:errorcluster)  [unwired: 8 in, 2 out]
        n160 = Index Array(array=w401, index=w372) -> (element=w397:T10)
        n161 = call "Interruptible Timer.vi"("error in (no error)"=w388, "Wait (s)"=1) -> ("error out"=w386:errorcluster)  [unwired: 7 in, 2 out]
        n162 = Unbundle By Name(w397) -> ("Gas"=w363:string, "ADC Gains"=w396:T11)
        n163 = call "Control Valve.vi"("Session Handle in"=w387, "Valves"=w392, "Energize?"=FALSE, "error in (no error)"=w386) -> ("Session Handle out"=w384:T14, "error out"=w385:errorcluster)  [unwired: 8 in, 2 out]
        n164 = Format Into String(format string="%s is now passing through the test fixture...", w363) -> (resulting string=w394:string)  [unwired: 2 in, 1 out]
        n165 = call "Set ADC Gain.vi"("Session Handle in"=w384, "ADC Gains"=w396, "error in (no error)"=w385) -> ("error out"=w376:errorcluster)  [unwired: 10 in, 2 out]
        n166 = call "Write to Message Log.vi"("error in (no error)"=w376, "Message"=w394) -> ("error out"=w366:errorcluster)  [unwired: 9 in]
        n167 = call "File Tracker.vi"("Gas"=w363, "Command"="new gas", "error in (no error)"=w366) -> ("error out"=w365:errorcluster)  [unwired: 7 in, 1 out]
        n168 = local read "PAS Temp"() -> (w367:dbl)
        n169 = local read "Moisture"() -> (w368:dbl)
        n170 = local read "Pressure"() -> (w369:dbl)
        n171 = local read "PPM"() -> (w370:dbl)
        n172 = Bundle By Name(cluster=w402, "Samples"=w371, "Gas"=w363, "PPM"=w370, "Moisture"=w368, "Pressure"=w369, "Temp"=w367) -> (w400:T16)
        n173 = call "Write to Message Log.vi"("error in (no error)"=w365, "Message"="Gas Stabilized. Starting Filter Rotations...") -> ("error out"=w381:errorcluster)  [unwired: 9 in]
        n174 = Bundle By Name(cluster=w399, "Test Info"=w400) -> (w398:T19)
      }
      frame "wait mix" {
        # "1, Check if all gases are done -> go to test done \n2. Check if current gas is OK to go ahead -> start mix\n                                                               ELSE -> wait mix"
        n175 = Unbundle By Name(w408) -> ("Test Config"=w404:T9)
        n176 = call "Test Tracker.vi"("Command"="check done", "error in (no error)"=w409, "Test Config"=w404) -> ("error out"=w405:errorcluster, "All Done?"=w406:bool)  [unwired: 5 in, 2 out]
        n177 = case shown="False" w406 {
          tunnel: [w419 "test done"] -> w410
          tunnel: w405 -> [w417 w426]
          tunnel: w404 -> [w416 _]
          tunnel: [w412 w426] -> w403
          frame False {
            # "IF current GAS = Gas Offered\n&& Gas is Stable && Time remaining is enough\n&& PPM matches in tolerance\ngo to start mix"
            n178 = local read "PPM"() -> (w414:dbl)
            n179 = local read "Gas"() -> (w415:string)
            n180 = call "Test Tracker.vi"("Command"="check gas", "error in (no error)"=w417, "PPM"=w414, "Gas Name"=w415, "Test Config"=w416) -> ("error out"=w412:errorcluster, "Proceed?"=w411:bool)  [unwired: 3 in, 2 out]
            n181 = local read "Time Remaining"() -> (w425:u32)
            n182 = local read "Gas Stable?"() -> (w424:bool)
            n183 = Greater?(x=w425, y=u32 900) -> (0:w423:bool)
            n184 = Compound Arithmetic op=AND(w411, w424, w423) -> (w422:bool)
            n185 = Select(t="Flush", s=w422, f="wait mix") -> (s? t:f=w419:string)
          }
          frame True {
          }
        }
      }
      frame "filter" {
        # "1. Check if Filter Sequence List is Done - > start a new mix\n2. If not, go to filter position\n3. Wait to settle"
        n186 = Unbundle By Name(w435) -> ("Test Config"=w432:T9, "Test Info"=w436:T16, "Test Config.Filter Sequences"=w442:T12[], "Test Info.Filter Counter"=w441:u16, "Test Config.Filter Time"=w437:u16, "PAS"=w438:T14)
        n187 = local read "PPM"() -> (w428:dbl)
        n188 = local read "Gas"() -> (w429:string)
        n189 = call "Test Tracker.vi"("Command"="valid check", "PPM"=w428, "Gas Name"=w429, "Test Config"=w432) -> ("Proceed?"=w431:bool)  [unwired: 4 in, 3 out]
        n190 = Array Size(array=w442) -> (size(s)=w445:i32)
        n191 = Greater?(x=w445, y=w441) -> (0:w444:bool)
        n192 = case shown="True" w431 {
          tunnel: w444 -> [_ w458]
          tunnel: w443 -> [w448 w457]
          tunnel: w442 -> [_ w456]
          tunnel: w441 -> [_ w455]
          tunnel: ["abort test" ("Error String") w454] -> w440
          tunnel: [w448 w453] -> w439
          tunnel: w438 -> [_ w452]
          tunnel: w437 -> [_ w451]
          tunnel: w436 -> [_ w450]
          tunnel: [_ w449] -> w433
          frame False {
            n193 = One Button Dialog(message="Error: The gas currently being distributed by the master is not the gas or at the correct PPM that is being tested by this unit. ") -> ()  [unwired: 1 in, 1 out]
          }
          frame True {
            n194 = case shown="False" w458 {
              tunnel: w457 -> [w462 w485]
              tunnel: w456 -> [_ w491]
              tunnel: w455 -> [_ w490]
              tunnel: [w460 w478] -> w453
              tunnel: ["wait mix" ("Error String") "record data" ("Error String")] -> w454
              tunnel: w452 -> [_ w488]
              tunnel: w451 -> [_ w477]
              tunnel: w450 -> [w469 w486]
              tunnel: [w470 w486] -> w449
              frame False {
                # "Make sure the gas tracker\nrecords this gas as done"
                # "1. Increment Gas Counter\n2. Reset Filter Counter"
                n195 = Unbundle By Name(w469) -> ("Gas Counter"=w468:u16)
                n196 = call "Write to Message Log.vi"("error in (no error)"=w462, "Message"="Gas Finished! Waiting for next gas...") -> ("error out"=w463:errorcluster)  [unwired: 9 in]
                n197 = Increment(x=w468) -> (x+1=w467:u16)
                n198 = Bundle By Name(cluster=w469, "Gas Counter"=w467, "Filter Counter"=u16 0) -> (w470:T16)
                n199 = call "Test Tracker.vi"("Command"="gas done", "error in (no error)"=w463) -> ("error out"=w461:errorcluster, "Gas Index"=w459:i32)  [unwired: 6 in, 2 out]
                n200 = call "Update Gas Status.vi"("error in (no error)"=w461, "index (row)"=w459) -> ("error out"=w460:errorcluster)  [unwired: 9 in]
              }
              frame True {
                n201 = Index Array(array=w491, index=w490) -> (element=w489:T12)
                n202 = Unbundle By Name(w489) -> ("Filter"=w482:u8, "Phase"=w474:dbl)
                n203 = Format Into String(format string="Go to Position #%d" ("initial string"), w482) -> (resulting string=w484:string)  [unwired: 2 in, 1 out]
                n204 = local write "Filter Position"(w482) -> ()
                n205 = call "Write to Message Log.vi"("error in (no error)"=w485, "Message"=w484) -> ("error out"=w483:errorcluster)  [unwired: 9 in]
                n206 = call "Filter Wheel Position Test.vi"("error in (no error)"=w483, "Position"=w482, "Session Handle in"=w488) -> ("error out"=w475:errorcluster, "Session Handle out"=w476:T14)  [unwired: 6 in, 1 out]
                n207 = call "Set Carrier Phase.vi"("Session Handle in"=w476, "Phase"=w474, "error in (no error)"=w475) -> ("Session Handle out"=w472:T14, "error out"=w473:errorcluster)  [unwired: 10 in, 1 out]
                n208 = call "Write to Message Log.vi"("error in (no error)"=w473, "Message"="Position Reached. Waiting for ADC to settle..." ("initial string")) -> ("error out"=w480:errorcluster)  [unwired: 9 in]
                n209 = call "Wait ADC Measurement.vi"("Wait (s)"=w477, "error in (no error)"=w480, "Session Handle in"=w472) -> ("error out"=w478:errorcluster)  [unwired: 5 in, 3 out]
              }
            }
          }
        }
        n210 = Bundle By Name(cluster=w435, "Test Info"=w433) -> (w434:T19)
      }
      frame "Flush" {
        n211 = call "Write to Message Log.vi"("error in (no error)"=w497, "Message"="Flushing gas for 300 seconds.") -> ("error out"=w496:errorcluster)  [unwired: 9 in]
        n212 = flat-sequence {
          tunnel: w496 -> [w501]
          tunnel: [w501] -> w494
          frame #0 {
            n213 = Wait (ms)(milliseconds to wait=u32 300000) -> ()  [unwired: 1 out]
          }
        }
        n214 = call "Write to Message Log.vi"("error in (no error)"=w494, "Message"="Gas flush finished.") -> ("error out"=w493:errorcluster)  [unwired: 9 in]
      }
      frame "record data" {
        # "1. Set Phase\n2. Obtain Readings\n3. Perform Mean and Avg\n4. Go to Record Result"
        n215 = call "Write to Message Log.vi"("error in (no error)"=w516, "Message"="Filter Settled. Taking Readings...") -> ("error out"=w503:errorcluster)  [unwired: 9 in]
        n216 = Unbundle By Name(w520) -> ("Test Info"=w518:T16, "Test Config.Filter Sequences"=w524:T12[], "Test Info.Filter Counter"=w525:u16, "Test Config.Samples"=w514:u16, "Test Config.A-D Settle"=w522:u16, "PAS"=w504:T14)
        n217 = Index Array(array=w524, index=w525) -> (element=w523:T12)
        n218 = Unbundle By Name(w523) -> ("Filter"=w508:u8, "Phase"=w507:dbl)
        n219 = Decrement(x=w514) -> (x-1=w513:u16)
        n220 = for {
          N: w514 -> [_]
          shift-right: [w531] -> _
          shift-left: w504 -> [w535]
          shift-right: [w533] -> w512
          shift-left: w503 -> [w536]
          tunnel: w522 -> [w532]
          tunnel: w513 -> [w530]
          tunnel: [w527] -> w502 mode=indexing
          i -> [w529]
          stop <- w526 stop-if-true
          n221 = call "Read ADC.vi"("Session Handle in"=w535, "error in (no error)"=w536) -> ("Session Handle out"=w531:T14, "ADC"=w527:dbl, "error out"=w534:errorcluster)  [unwired: 9 in, 2 out]
          n222 = Subtract(x=w530, y=w529) -> (x-y=w528:i32)
          n223 = local write "Samples Left"(w528) -> ()
          n224 = call <userlib>:"Wait (ms)__ogtk.vi"("error in (no error)"=w534, "milliseconds to wait"=w532) -> ("error out"=w533:errorcluster)  [unwired: 8 in, 1 out]
          n225 = shared-variable ".\\Abort.lvlib\\Abort"() -> (w526:bool)  [unwired: 1 in, 1 out]
        }
        n226 = call <vilib>:"Std Deviation and Variance.vi"("X"=w502) -> ("mean"=w506:dbl, "standard deviation"=w505:dbl)  [unwired: 1 in, 1 out]
        n227 = Select(t="Error", s=w512, f="Success") -> (s? t:f=w509:string)
        n228 = Bundle By Name(cluster=w518, "Notes"=w509, "Filter"=w508, "Phase"=w507, "Mean"=w506, "STD"=w505) -> (w517:T16)
        n229 = Bundle By Name(cluster=w520, "Test Info"=w517) -> (w519:T19)
      }
      frame "record result" {
        # "1. Write result to Test Result\n2. Increment Filter\n3. Go to Filter"
        n230 = call "Write to Message Log.vi"("error in (no error)"=w546, "Message"="Readings Finished. Recording Result...") -> ("error out"=w540:errorcluster)  [unwired: 9 in]
        n231 = Unbundle By Name(w549) -> ("Results"=w543:T16[], "Test Info"=w538:T16, "Test Info.Filter Counter"=w541:u16, "Test Config.Samples"=w542:u16)
        n232 = call "File Tracker.vi"("Command"="write result", "error in (no error)"=w540, "Result"=w538) -> ("error out"=w539:errorcluster)  [unwired: 7 in, 1 out]
        n233 = local write "Samples Left"(w542) -> ()
        n234 = Increment(x=w541) -> (x+1=w544:u16)
        n235 = Build Array (concatenate)(w543, w538) -> (w545:T16[])
        n236 = Bundle By Name(cluster=w549, "Results"=w545, "Test Info.Filter Counter"=w544) -> (w548:T19)
      }
      frame "test done" {
        # "1. Initialize HW to turn off gas flow\n2 Call Calculation Engine\n3. Write PAS Values"
        n237 = call "Initialize Hardware.vi"("error in"=w555) -> ("error out"=w554:errorcluster)  [unwired: 10 in]
        n238 = call "File Tracker.vi"("Command"="close", "error in (no error)"=w554) -> ("error out"=w565:errorcluster, "File Contents"=w564:string)  [unwired: 8 in]
        n239 = Unbundle By Name(w569) -> ("PAS"=w568:T14)
        n240 = local write "Test"("Test Complete..." ("Test")) -> ()
        n241 = call "Calibrate.vi"("error in (no error)"=w565, "input"=w564) -> ("error out"=w563:errorcluster, "blob"=w561:u8[])  [unwired: 8 in]
        n242 = call "Write to Message Log.vi"("error in (no error)"=w563, "Message"="Writing Calibration Coefficients to PAS Board. This will take 2.5 minutes") -> ("error out"=w562:errorcluster)  [unwired: 9 in]
        n243 = call "File Tracker.vi"("Command"="write blob", "error in (no error)"=w562, "Blob"=w561) -> ("error out"=w559:errorcluster)  [unwired: 7 in, 1 out]
        n244 = call "Write Blob to PAS Board.vi"("Session Handle in"=w568, "Bytes to Write"=w561, "error in (no error)"=w559) -> ("error out"=w558:errorcluster)  [unwired: 11 in, 1 out]
        n245 = call "Write to Message Log.vi"("error in (no error)"=w558, "Message"="Write Complete!") -> ("error out"=w556:errorcluster)  [unwired: 9 in]
        n246 = call "Write to Message Log.vi"("error in (no error)"=w556, "Message"="Test Completed Sucessfully!") -> ("error out"=w552:errorcluster)  [unwired: 9 in]
        n247 = shared-variable ".\\Progress.lvlib\\Progress"(FALSE ("Progress"), error in=w552) -> (error out=w551:errorcluster)
      }
      frame "abort test" {
        w584 = FALSE ("Progress")
        # "1. Write Test Aborted to Message Log and Popup Dialog\n2. Init HW\n3. Turn Progress and Abort GV OFF"
        n248 = call "Write to Message Log.vi"("error in (no error)"=w580, "Message"="Test Aborted..." ("Test")) -> ("error out"=w581:errorcluster)  [unwired: 9 in]
        n249 = local write "Test"("Test Aborted..." ("Test")) -> ()
        n250 = call "Initialize Hardware.vi"("error in"=w581) -> ("error out"=w587:errorcluster)  [unwired: 10 in]
        n251 = shared-variable ".\\Progress.lvlib\\Progress"(w584, error in=w587) -> (error out=w583:errorcluster)
        n252 = shared-variable ".\\Abort.lvlib\\Abort"(w584) -> (error out=w582:errorcluster)  [unwired: 1 in]
        n253 = Merge Errors(w583, w582) -> (w574:errorcluster)
        n254 = call "File Tracker.vi"("Command"="close", "error in (no error)"=w574) -> ("error out"=w573:errorcluster)  [unwired: 8 in, 1 out]
        n255 = flat-sequence {
          tunnel: "Test Aborted!" ("Message") -> [w589]
          tunnel: w573 -> [w588]
          tunnel: [w588] -> w578
          frame #0 {
            n256 = One Button Dialog(message=w589) -> ()  [unwired: 1 in, 1 out]
          }
        }
        n257 = Unbundle By Name(w576) -> ("State"=w575:refnum<queue>)
        n258 = Flush Queue(queue=w575, error in (no error)=w578) -> (error out=w577:errorcluster)  [unwired: 2 out]
      }
    }
    n259 = Unbundle By Name(w100) -> ("State"=w101:refnum<queue>)
    n260 = Wait (ms)(milliseconds to wait=u32 500) -> ()  [unwired: 1 out]
    n261 = call "State Machine - Enqueue State.vi"("error in (no error)"=w108, "State"=w107, "Queue In"=w101) -> ("error out"=w109:errorcluster, "Queue Out"=w98:refnum<queue>)  [unwired: 7 in]
  }
  n262 = call "Obtain Session.vi"("Session  Name ()"="Snap", "error in (no error)"=w18) -> ("Session Handle"=w16:T24, "error out"=w17:errorcluster)  [unwired: 12 in]
  n263 = while {
    tunnel: w17 -> [w599]
    shift-right: [w595] -> _
    shift-left: w16 -> [w598]
    tunnel: [w596] -> _
    stop <- w600 stop-if-true
    n264 = call "Read Snapshot.vi"("Session Handle in"=w598, "error in (no error)"=w599) -> ("Session Handle out"=w595:T24, "Buffer"=w594:dbl[], "error out"=w596:errorcluster)  [unwired: 11 in]
    n265 = local read "exit"() -> (w600:bool)
    n266 = Index Array(array=w594) -> (element #1=→"Pressure":dbl, element #2=→"PAS Temp":dbl, element #3=→"PEL Temp":dbl, element #4=→"Leak Rate":dbl)  [unwired: 4 in]
    n267 = Wait (ms)(milliseconds to wait=u32 1000) -> ()  [unwired: 1 out]
  }
  n268 = while {
    tunnel: errorcluster {"status"=FALSE, "code"=0, "source"=""} ("error in (no error)") -> [w602]
    tunnel: [w601] -> _
    stop <- w603 stop-if-true
    n269 = event shown="[3] \"Manual\": Value Change" {
      selector: _ -> [_ _ _ _ _ _]
      dyn-events: _ -> [_ _ _ _ _ _]
      timeout: _ -> [_ _ _ _ _ _]
      tunnel: [_ w606 _ _ _ _] -> w603
      tunnel: w602 -> [w604 w607 w632 w656 w669 w685]
      tunnel: [w604 w608 w631 w652 w672 w684] -> w601
      event Timeout {
        n270 = event-data() -> ()  [unwired: 1 in, 3 out]
      }
      event Value Change {
        n271 = event-data() -> ()  [unwired: 1 in, 1 out]
        n272 = shared-variable ".\\Progress.lvlib\\Progress"() -> (w605:bool)  [unwired: 1 in, 1 out]
        n273 = case shown="False" w605 {
          tunnel: [w613 w628] -> w608
          tunnel: w607 -> [w612 w628]
          tunnel: [w609 FALSE] -> w606
          frame False {
            n274 = Two Button Dialog(message="Are you sure you would like to exit?") -> (T button?=w610:bool)  [unwired: 2 in]
            n275 = case shown="True" w610 {
              tunnel: [w614 w619] -> w613
              tunnel: w612 -> [w614 w618]
              tunnel: [_ TRUE] -> w609
              frame False {
              }
              frame True {
                n276 = shared-variable ".\\Exit.lvlib\\Exit"(TRUE ("Exit"), error in=w618) -> (error out=w617:errorcluster)
                n277 = Obtain Queue(name (unnamed)="Slave", element data type=variant, error in (no error)=w617) -> (queue out=w623:refnum<queue>, error out=w624:errorcluster)  [unwired: 2 in, 1 out]
                n278 = call "State Machine - Enqueue State.vi"("error in (no error)"=w624, "State"="exit", "Queue In"=w623) -> ("error out"=w621:errorcluster, "Queue Out"=w620:refnum<queue>)  [unwired: 7 in]
                n279 = Release Queue(queue=w620, error in (no error)=w621) -> (error out=w619:errorcluster)  [unwired: 1 in, 2 out]
              }
            }
          }
          frame True {
            n280 = One Button Dialog(message="Please abort currently running test if you wish to quit") -> ()  [unwired: 1 in, 1 out]
          }
        }
      }
      event Value Change {
        n281 = event-data() -> ()  [unwired: 1 in, 1 out]
        n282 = shared-variable ".\\Progress.lvlib\\Progress"() -> (w630:bool)  [unwired: 1 in, 1 out]
        n283 = case shown="False" w630 {
          tunnel: w632 -> [w639 w649]
          tunnel: [w640 w649] -> w631
          frame False {
            n284 = call "Request Serial Number.vi"("error in (no error)"=w639, "Serial Number"="PAS") -> ("error out"=w638:errorcluster, "Serial Number Out"=w636:string)  [unwired: 8 in]
            n285 = call "Request System Operator Name.vi"("error in (no error)"=w638) -> ("error out"=w637:errorcluster, "Operator"=w635:string)  [unwired: 9 in]
            n286 = Bundle("Serial Number Out"=w636, "Operator"=w635) -> (w634:T22)  [unwired: 1 in]
            n287 = Obtain Queue(name (unnamed)="Slave", element data type=variant, error in (no error)=w637) -> (queue out=w644:refnum<queue>, error out=w645:errorcluster)  [unwired: 2 in, 1 out]
            n288 = call "State Machine - Enqueue State.vi"("error in (no error)"=w645, "Data"=w634, "State"="init test", "Queue In"=w644) -> ("error out"=w642:errorcluster, "Queue Out"=w641:refnum<queue>)  [unwired: 6 in]
            n289 = Release Queue(queue=w641, error in (no error)=w642) -> (error out=w640:errorcluster)  [unwired: 1 in, 2 out]
          }
          frame True {
            n290 = One Button Dialog(message="Test already in progress. Please wait until the test is over, or abort the test and start a new one.") -> ()  [unwired: 1 in, 1 out]
          }
        }
      }
      event Value Change {
        n291 = event-data() -> ()  [unwired: 1 in, 2 out]
        n292 = call "Get User Configuration File.vi"("error in (no error)"=w656) -> ("error out"=w655:errorcluster, "Config"=w651:T25)  [unwired: 9 in]
        n293 = Unbundle By Name(w651) -> ("Password"=w650:string)
        n294 = disable-structure shown="Enabled" {
          disable-tunnel: w655 -> [w660 w662]
          disable-tunnel: [w659 w662] -> w654
          disable-tunnel: [w658 TRUE ("Success?")] -> w653
          disable-tunnel: w650 -> [w657 _]
          frame Disabled {
            n295 = call "Get Password From User.vi"("error in"=w660, "password"=w657) -> ("error out"=w659:errorcluster, "Success?"=w658:bool)  [unwired: 8 in]
          }
          frame Enabled {
          }
        }
        n296 = case shown="True" w653 {
          tunnel: w654 -> [w663 w665]
          tunnel: [w663 w665] -> w652
          frame False {
            n297 = One Button Dialog(message="Invalid Password!" ("Message")) -> ()  [unwired: 1 in, 1 out]
          }
          frame True {
            n298 = call "Manual Mode.vi"() -> ()  [unwired: 12 in]
          }
        }
      }
      event Value Change {
        n299 = event-data() -> ()  [unwired: 1 in, 1 out]
        n300 = call "Read Configuration File.vi"("error in (no error)"=w669) -> ("error out"=w668:errorcluster, "User Config"=w667:T25)  [unwired: 9 in]
        n301 = Unbundle By Name(w667) -> ("Password"=w666:string)
        n302 = disable-structure shown="Enabled" {
          disable-tunnel: [w676 w678] -> w671
          disable-tunnel: [w675 TRUE ("Success?")] -> w670
          disable-tunnel: w668 -> [w674 w678]
          disable-tunnel: w666 -> [w673 _]
          frame Disabled {
            n303 = call "Get Password From User.vi"("error in"=w674, "password"=w673) -> ("error out"=w676:errorcluster, "Success?"=w675:bool)  [unwired: 8 in]
          }
          frame Enabled {
          }
        }
        n304 = case shown="True" w670 {
          tunnel: [w680 w681] -> w672
          tunnel: w671 -> [w680 w682]
          frame False {
            n305 = One Button Dialog(message="Invalid Password!" ("Message")) -> ()  [unwired: 1 in, 1 out]
          }
          frame True {
            n306 = call "Configure Slave Test.vi"("error in (no error)"=w682) -> ("error out"=w681:errorcluster)  [unwired: 10 in]
          }
        }
      }
      event Value Change {
        n307 = event-data() -> ()  [unwired: 1 in, 1 out]
        n308 = shared-variable ".\\Progress.lvlib\\Progress"() -> (w683:bool)  [unwired: 1 in, 1 out]
        n309 = case shown="True" w683 {
          tunnel: w685 -> [w687 w691]
          tunnel: [w687 w690] -> w684
          frame False {
            n310 = One Button Dialog(message="No Test in Progress!") -> ()  [unwired: 1 in, 1 out]
          }
          frame True {
            n311 = Two Button Dialog(message="Are you sure you would like to abort the test?") -> (T button?=w689:bool)  [unwired: 2 in]
            n312 = case shown="True" w689 {
              tunnel: w691 -> [w692 w704]
              tunnel: [w692 w694] -> w690
              frame False {
              }
              frame True {
                n313 = shared-variable ".\\Abort.lvlib\\Abort"(TRUE ("Abort"), error in=w704) -> (error out=w696:errorcluster)
                n314 = Obtain Queue(name (unnamed)="Slave", element data type=variant, error in (no error)=w696) -> (queue out=w699:refnum<queue>, error out=w700:errorcluster)  [unwired: 2 in, 1 out]
                n315 = call "State Machine - Enqueue State.vi"("Front?"=TRUE, "error in (no error)"=w700, "State"="abort test", "Queue In"=w699) -> ("error out"=w698:errorcluster, "Queue Out"=w697:refnum<queue>)  [unwired: 6 in]
                n316 = Release Queue(queue=w697, error in (no error)=w698) -> (error out=w694:errorcluster)  [unwired: 1 in, 2 out]
              }
            }
          }
        }
      }
    }
  }
  n317 = Release Queue(queue=w13, error in (no error)=w21) -> ()  [unwired: 1 in, 3 out]
  n318 = disable-structure shown="RUN_TIME_ENGINE==False, Default" {
    disable-tunnel: w13 -> [_ _]
    frame condition #0 {
      n319 = Quit LabVIEW() -> ()  [unwired: 1 in]
    }
    frame condition #1 (active) {
    }
  }
